vi "Write Configuration.vi"(8 "error in (no error)":errorcluster, 10 "Configuration":T1, 11 "ADAS PE Template Controller in":refnum<class "PE Controller.lvclass">) -> (0 "error out":errorcluster, 3 "ADAS PE Template Controller out":refnum<class "PE Controller.lvclass">)   [LabVIEW 2020, in "ADAS PE Template.lvlib" / "PE Controller.lvclass"]
doc: "<b>Write Configuration</b>\nWrites the configuration information to the plugin controller class data."
uses:
  PE Controller.lvclass
  PE/Configuration.ctl
  PE Controller.lvclass/PE Controller.ctl
  PE/ADAS PE Template.lvclass
panel:
  # "#via_ignore"
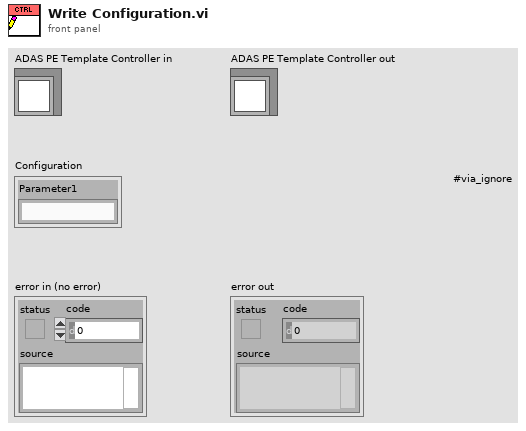
[diagram p1: front panel]
types:
  T1 = typedef "ADAS PE Template.lvlib/ADAS PE Template.lvclass/Configuration.ctl" = cluster{"Parameter1":string}
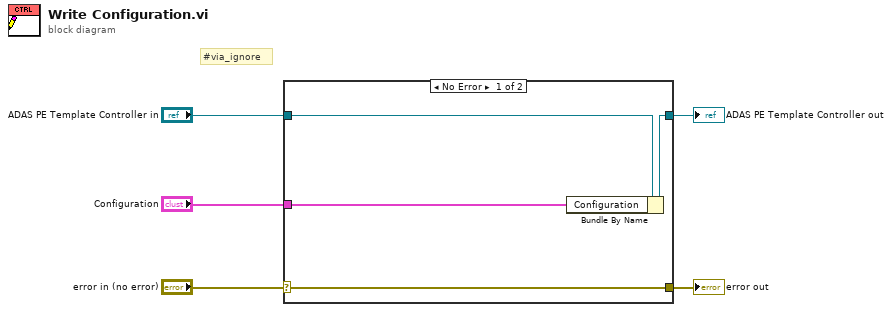
[diagram p0: block diagram]
diagram:
  # "#via_ignore"
  n1 = case shown="No Error" "error in (no error)" {
    selector: "error in (no error)" -> [w9 w10]
    tunnel: [w9 w10] -> w4
    tunnel: [w7 w11] -> w2
    tunnel: "ADAS PE Template Controller in" -> [w8 w11]
    tunnel: "Configuration" -> [w6 _]
    frame No Error {
      n2 = Bundle By Name(cluster=w8, "Configuration"=w6) -> (w7:refnum<class "PE Controller.lvclass">)
    }
    frame Error {
    }
  }
  "error out" <- w4
  "ADAS PE Template Controller out" <- w2
